vi "LIFA_test_2.vi"() -> ()   [LabVIEW 2011]
uses:
  <vilib>/LabVIEW Interface for Arduino/LabVIEW Interface for Arduino.lvlib
panel:
  out "Chart":sgl(graph)
  in  "stop":bool
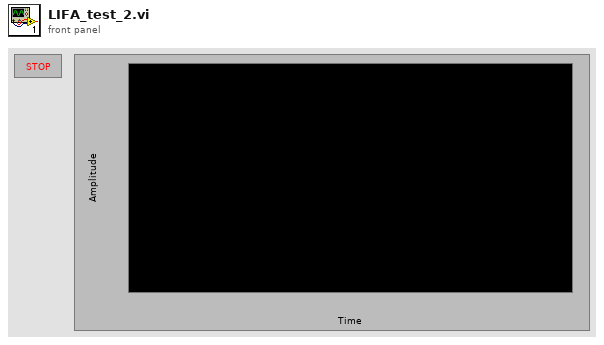
[diagram p1: front panel]
types:
  T1 = typedef "LabVIEW Interface for Arduino.lvlib/Arduino Resource.ctl" = cluster{"VISA resource":refnum<visa-resource-name>, "Board Type":T2, "Connection Type":enum8{"USB / Serial"}, "Bytes Per Packet (15)":u8}
  T2 = typedef "LabVIEW Interface for Arduino.lvlib/Board Type.ctl" = enum16{"Uno", "Mega 2560"}
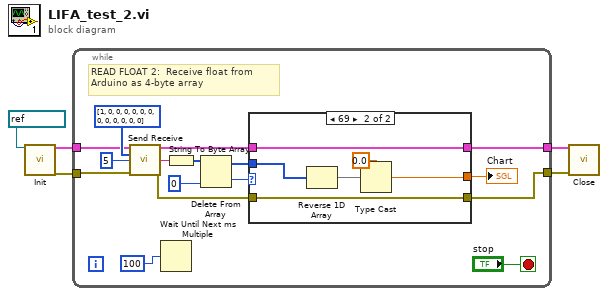
[diagram p0: block diagram]
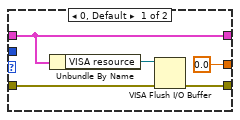
[diagram p2: hidden frame]
diagram:
  n1 = call <vilib>:"Init.vi"("VISA resource"=refnum<visa-resource-name> "COM4") -> ("Arduino Resource"=w5:T1, "error out"=w4:errorcluster)  [unwired: 17 in]
  n2 = while {
    tunnel: w5 -> [w17]
    tunnel: w4 -> [w16]
    tunnel: [w8] -> w2
    tunnel: [w6] -> w1
    stop <- "stop" stop-if-true
    # "READ FLOAT 2:  Receive float from Arduino as 4-byte array"
    n3 = call <vilib>:"Send Receive.vi"("Arduino Resource"=w17, "Data"=u8[] [1, 0, 0, 0, 0, 0, 0, 0, 0, 0, 0, 0, 0], "Bytes To Read (0)"=u8 5, "error in"=w16) -> ("Arduino Resource"=w7:T1, "Read Buffer"=w15:string, "error out"=w9:errorcluster)  [unwired: 9 in]
    n4 = Wait Until Next ms Multiple(millisecond multiple=u32 100 ("millisecond timer value")) -> ()  [unwired: 1 out]
    n5 = String To Byte Array(string=w15) -> (unsigned byte array=w14:u8[])
    n6 = Delete From Array(array=w14, index=0) -> (deleted portion=w12:u8, array with subset deleted=w11:u8[])  [unwired: 1 in]
    n7 = case shown="69" w12 {
      tunnel: w11 -> [_ w30]
      tunnel: [sgl 0.0 w29] -> w10
      tunnel: w9 -> [w25 w28]
      tunnel: [w24 w28] -> w8
      tunnel: w7 -> [w22 w27]
      tunnel: [w22 w27] -> w6
      frame 0, Default {
        n8 = Unbundle By Name(w22) -> ("VISA resource"=w26:refnum<visa-resource-name>)
        n9 = VISA Flush I/O Buffer(VISA resource name=w26, error in (no error)=w25) -> (error out=w24:errorcluster)  [unwired: 1 in, 1 out]
      }
      frame 105 {
        n10 = Reverse 1D Array(array=w30) -> (reversed array=w32:u8[])
        n11 = Type Cast(type=sgl 0.0, x=w32) -> (*(type *) &x=w29:sgl)
      }
    }
    "Chart" <- w10
  }
  n12 = call <vilib>:"Close.vi"("Arduino Resource"=w1, "error in"=w2) -> ()  [unwired: 13 in, 1 out]
